vi "SMS Analysis Get Image Type.vi"() -> (8 "Channel Code":u8)   [LabVIEW 2020]
uses:
  <vilib>/Utility/miscctls.llb/LVPointTypeDef.ctl
panel:
  in  "Cancel":bool
  in  "Quit":bool
  in  "Image Type":u8(ring) items=["Unknown", "Single Color - Left", "Single Color - Right", "Two Color Simultaneous", "Two Color SF"]
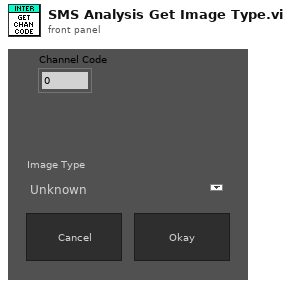
[diagram p1: front panel]
types:
  T1 = enum16{"Always On", "Always Off", "Off While Running"}
  T2 = typedef "LVPointTypeDef.ctl" = cluster{"Horizontal":i16, "Vertical":i16}
  T3 = typedef "LVRectTypeDef.ctl" = cluster{"Left":i16, "Top":i16, "Right":i16, "Bottom":i16}
  T4 = typedef "LVBoundsTypeDef.ctl" = cluster{"Width":u32, "Height":u32}
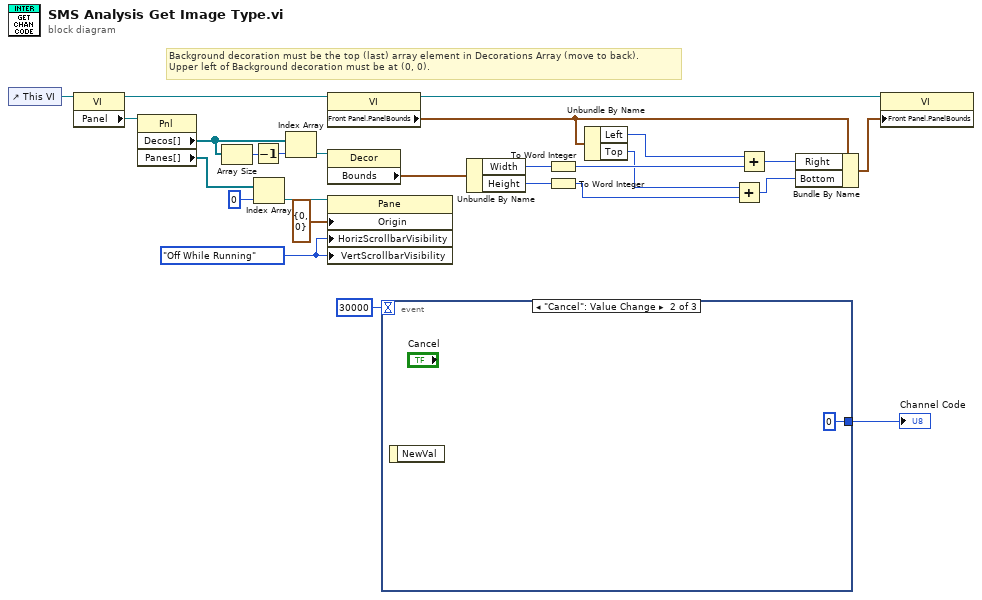
[diagram p0: block diagram]
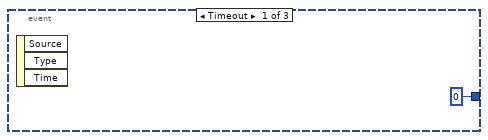
[diagram p2: hidden frame]
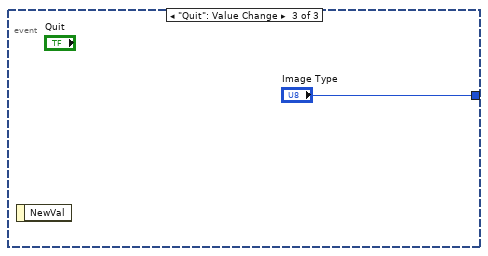
[diagram p3: hidden frame]
diagram:
  w14 = T1."Off While Running" ("Vertical Scrollbar Visibility")
  # "Background decoration must be the top (last) array element in Decorations Array (move to back).\nUpper left of Background decoration must be at (0, 0)."
  n1 = control-ref of="This VI"() -> (w7:refnum<vi>)
  n2 = property class="VI"(reference=w7) -> (reference out=w15:refnum<vi>, "Panel"=w8:refnum<vi>)  [unwired: 1 in, 1 out]
  n3 = property class="Pnl"(reference=w8) -> ("Decos[]"=w6:refnum<vi>[], "Panes[]"=w11:refnum<vi>[])  [unwired: 1 in, 2 out]
  n4 = Array Size(array=w6) -> (size(s)=w4:i32)
  n5 = Decrement(x=w4) -> (x-1=w5:i32)
  n6 = Index Array(array=w11, index=0) -> (element=w10:refnum<vi>)
  n7 = Index Array(array=w6, index=w5) -> (element=w13:refnum<vi>)
  n8 = property class="VI"(reference=w15) -> (reference out=w17:refnum<vi>, "Front Panel.PanelBounds"=w18:T3)  [unwired: 1 in, 1 out]
  n9 = property class="Decor"(reference=w13) -> ("Bounds"=w16:T4)  [unwired: 1 in, 2 out]
  n10 = property class="Pane"(reference=w10, "Origin"=T2 {"Horizontal"=0, "Vertical"=0}, "HorizScrollbarVisibility"=w14, "VertScrollbarVisibility"=w14) -> ()  [unwired: 1 in, 2 out]
  n11 = event shown="[1] \"Cancel\": Value Change" {
    selector: _ -> [_ _ _]
    dyn-events: _ -> [_ _ _]
    timeout: 30000 -> [_ _ _]
    tunnel: [u8 0 ("Image Type") u8 0 ("Image Type") "Image Type"] -> w26
    event Timeout {
      n12 = event-data() -> ()  [unwired: 1 in, 3 out]
    }
    event "Cancel": Value Change {
      n13 = event-data() -> ()  [unwired: 1 in, 1 out]
    }
    event "Quit": Value Change {
      n14 = event-data() -> ()  [unwired: 1 in, 1 out]
    }
  }
  "Channel Code" <- w26
  n15 = Unbundle By Name(w16) -> ("Width"=w21:u32, "Height"=w24:u32)
  n16 = To Word Integer(number=w21) -> (16bit integer=w23:i16)
  n17 = To Word Integer(number=w24) -> (16bit integer=w2:i16)
  n18 = Unbundle By Name(w18) -> ("Left"=w20:i16, "Top"=w3:i16)
  n19 = Add(x=w3, y=w2) -> (x+y=w1:i16)
  n20 = Add(x=w20, y=w23) -> (x+y=w22:i16)
  n21 = Bundle By Name(cluster=w18, "Right"=w22, "Bottom"=w1) -> (w19:T3)
  n22 = property class="VI"(reference=w17, "Front Panel.PanelBounds"=w19) -> ()  [unwired: 1 in, 2 out]
